vi "340 Install curve.vi"() -> ()   [LabVIEW 2014]
uses:
  <vilib>/Utility/file.llb/Read From Spreadsheet File (DBL).vi
panel:
  in  "String":string="arkady 21 X86677 0 bbb 2\n0.25801\t4.45375E6\n0.27737\t2.62566E6\n0.29819\t1.60932E6\n0.32056\t1.02188E6\n0.34462\t670072.53973\n0.37048\t452436.26441\n0.39828\t313746.29687\n0.42817\t222930.45266\n0.4603\t161962.57325\n0.49484\t120085.41205\n0.53198\t90709.71558\n0.5719\t69700.59447\n0.61482\t54404.56821\n0.66096\t43083.06528\n0.71055\t34574.75489\n0.76388\t28089.82505\n0.8212\t23082.06075\n0.88283\t19167.7648\n0.94908\t16073.44039\n1.0203\t13601.46108\n1.09686\t11607.18615\n1.17917\t9983.47778\n1.26766\t8650.07908\n1.36279\t7546.23042\n1.46506\t6625.47288\n1.575\t5851.94795\n1.69319\t5197.73327\n1.82026\t4640.90424\n1.95685\t4164.10967\n2.1037\t3753.51517\n2.26157\t3398.01249\n2.43128\t3088.6226\n2.61373\t2818.04165\n2.80988\t2580.29273\n3.02074\t2370.45687\n3.24742\t2184.46393\n3.49112\t2018.92875\n3.7531\t1871.02208\n4.03474\t1738.36829\n4.33752\t1618.96369\n4.66302\t1511.11116\n5.01295\t1413.36735\n5.38913\t1324.49994\n5.79355\t1243.45283\n6.22831\t1169.31762\n6.6957\t1101.31025\n7.19817\t1038.75164\n7.73834\t981.0517\n8.31905\t927.69602\n8.94333\t878.23474\n9.61446\t832.27325\n10.33596\t789.46439\n11.1116\t749.50181\n11.94545\t712.1145\n12.84187\t677.06201\n13.80556\t644.13049\n14.84156\t613.12931\n15.95532\t583.88816\n17.15265\t556.25465\n18.43983\t530.09215\n19.82361\t505.27808\n21.31123\t481.70232\n22.91048\t459.26597\n24.62975\t437.8802\n26.47804\t417.46531\n28.46502\t397.94989\n30.60112\t379.27007\n32.89751\t361.36896\n35.36624\t344.19602\n38.02022\t327.70658\n40.87336\t311.86138\n43.94061\t296.62609\n47.23804\t281.97099\n50.78292\t267.87048\n54.59381\t254.3027\n58.69068\t241.2492\n63.095\t228.69448\n67.82982\t216.62562\n72.91996\t205.0319\n78.39208\t193.90438\n84.27485\t183.23555\n90.59907\t173.01889\n97.39788\t163.24857\n104.70689\t153.91906\n112.56439\t145.02481\n121.01154\t136.55996\n130.09259\t128.51808\n139.8551\t120.89196\n150.35022\t113.6734\n161.63293\t106.85306\n173.76232\t100.42039\n186.80193\t94.36354\n200.82007\t88.66931\n215.89018\t83.32316\n232.09118\t78.30923\n249.50796\t73.61033\n268.23174\t69.20805\n288.36061\t65.08274\n310\t61.21363\n"
  in  "VISA resource name":refnum<visa-resource-name>
  in  "Curve (21)":dbl=21.0 min=21.0 max=60.0 step=1.0
  out "error out":errorcluster
  in  "error in (no error)":errorcluster
  in  "file path (dialog if empty)":path
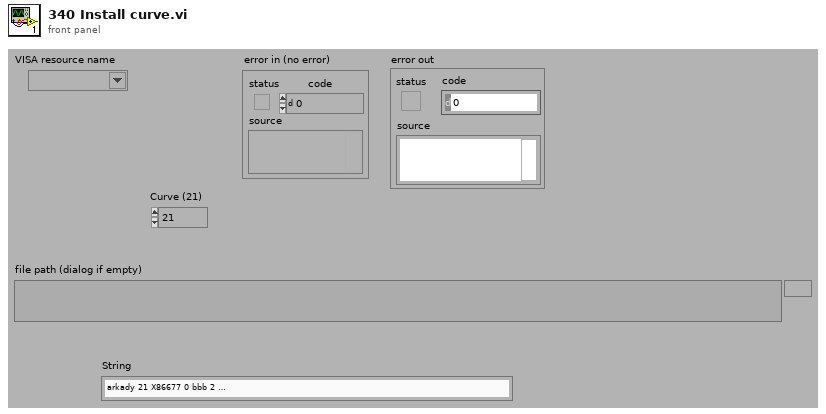
[diagram p1: front panel]
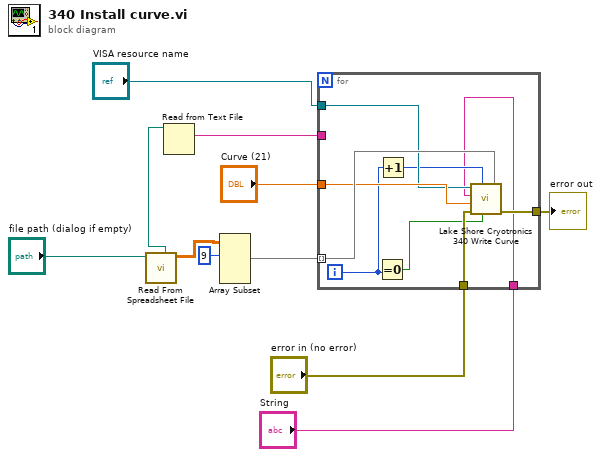
[diagram p0: block diagram]
diagram:
  n1 = call-poly <vilib>:"Read From Spreadsheet File.vi"("file path (dialog if empty)"="file path (dialog if empty)") -> ("all rows"=w9:dbl[][], "new file path (Not A Path if cancelled)"=w4:path)  [unwired: 6 in, 3 out]
  n2 = Read from Text File(file (use dialog)=w4) -> (text=w3:string)  [unwired: 3 in, 3 out]
  n3 = Array Subset(array=w9, index (row)=9 ("index")) -> (w8:dbl[][])  [unwired: 3 in]
  n4 = for {
    tunnel: w8 -> [w20] mode=indexing
    tunnel: "error in (no error)" -> [w19]
    tunnel: [w18] -> w6
    tunnel: "Curve (21)" -> [w17]
    tunnel: w3 -> [_]
    tunnel: "VISA resource name" -> [w16]
    tunnel: "String" -> [w12]
    i -> [w14]
    n5 = Equal To 0?(x=w14) -> (x = 0?=w15:bool)
    n6 = Increment(x=w14) -> (x+1=w13:i32)
    n7 = call "Lake Shore Cryotronics 340 Write Curve.vi"("Array"=w20, "Write Curve\nHeader (F: Don't Write Header)"=w15, "index"=w13, "error in (no error)"=w19, "Curve (21)"=w17, "String"=w12, "VISA resource name"=w16) -> ("error out"=w18:errorcluster)  [unwired: 2 in]
  }
  "error out" <- w6
